vi "Create.vi"   [LabVIEW 2020, in "LINX Server.lvclass"]
uses:
  LINX Server.lvclass
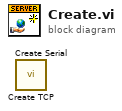
[diagram p0: block diagram]
diagram:
  n1 = call "Create TCP.vi"() -> ()  [unwired: 10 in, 2 out]
  n2 = call "Create Serial.vi"() -> ()  [unwired: 10 in, 2 out]
